vi "PDF Protokoll EPA1065_307.vi"(8 "error in (no error)":errorcluster caption="Fehler (Eingang, kein Fehler)") -> (0 "error out":errorcluster caption="Fehler (Ausgang)")   [LabVIEW 2020, in "Linearisierung v2.lvlib" / "Protokoll.lvlib"]
uses:
  Protokoll.lvlib
  EPA Ausgabetabelle.ctl
  AktivArray.ctl
  AktivButton.ctl
  Aktion Lin Daten aufarbeiten.ctl
  EPA1065-307/Aktion FGV Auswertung sammeln.ctl
  Seiten/FT-IR/FGV FT-IR Aktionen.ctl
  Seiten/System Einstellungen V2/Aktioen FGV System Konstanten.ctl
  Seiten/FT-IR/FGV FT-IR Gasliste Aktionen.ctl
  Seiten/System Einstellungen V2/Aktion FGV SystemEinstellungenV2.ctl
  Gasteiler/Aktionen FGV Gasteiler Daten.ctl
  <vilib>/Utility/miscctls.llb/LVPrintingMarginsTypeDef.ctl
  Linearisierung v2.lvlib
  EPA1065-307/Linearity verification 1065-307.lvlib
  Allgemein/allgemeine Sub-VIs.lvlib
  Seiten/FT-IR/FT-IR.lvlib
  Seiten/System Einstellungen V2/System Einstellungen V2.lvlib
  Gasteiler/Gasteiler.lvlib
panel:
  out "Serial number GT":string caption="Seriennummer:"
  out "Accuracy:":string caption="Genauigkeit:"
  out "Gas Bottle Nr.:":string caption="Gasflaschen Nr.:"
  out "Methode (Recipe):":string caption="Methode (Rezept):"
  out "Date & Time:":string caption="Datum & Zeit:"
  out "Versa Serial number:":string caption="Seriennummer:"
  out "Anlage:":string
  out "Serial number:":string caption="Seriennummer:"
  out "Messgerät:":string
  out "XY-Graph EPA":cluster{dbl[], dbl[]}[](graph) caption="XY-Graph"
  out "Aktiv":T1
  out "EPA Ausgabetabelle":T3
  out "Ergebnis:":string
  out "Konzentration:":string
  out "Komponente:":string
  out "Bearbeiter:":string
  out "Gasteiler:":string
  out "EPA Auswertung":string[][](table) caption="Evaluation"
  # "Linearity Check EPA § 1065.307"
  # "Linearity detection §1065.307"
  # "Description of the limits"
  # "Slope (a1) value between 0,99-1,01"
  # "Intercept (a0)"
  # "laboratory: Value <= 0,5% of the gas concentration"
  # "field: Value <= 1% of the gas concentration"
  # "Coefficient of determination (R²) Value >= 0,998"
  # "standard error of estimate (SEE) Value <= 1% of the gas concentration"
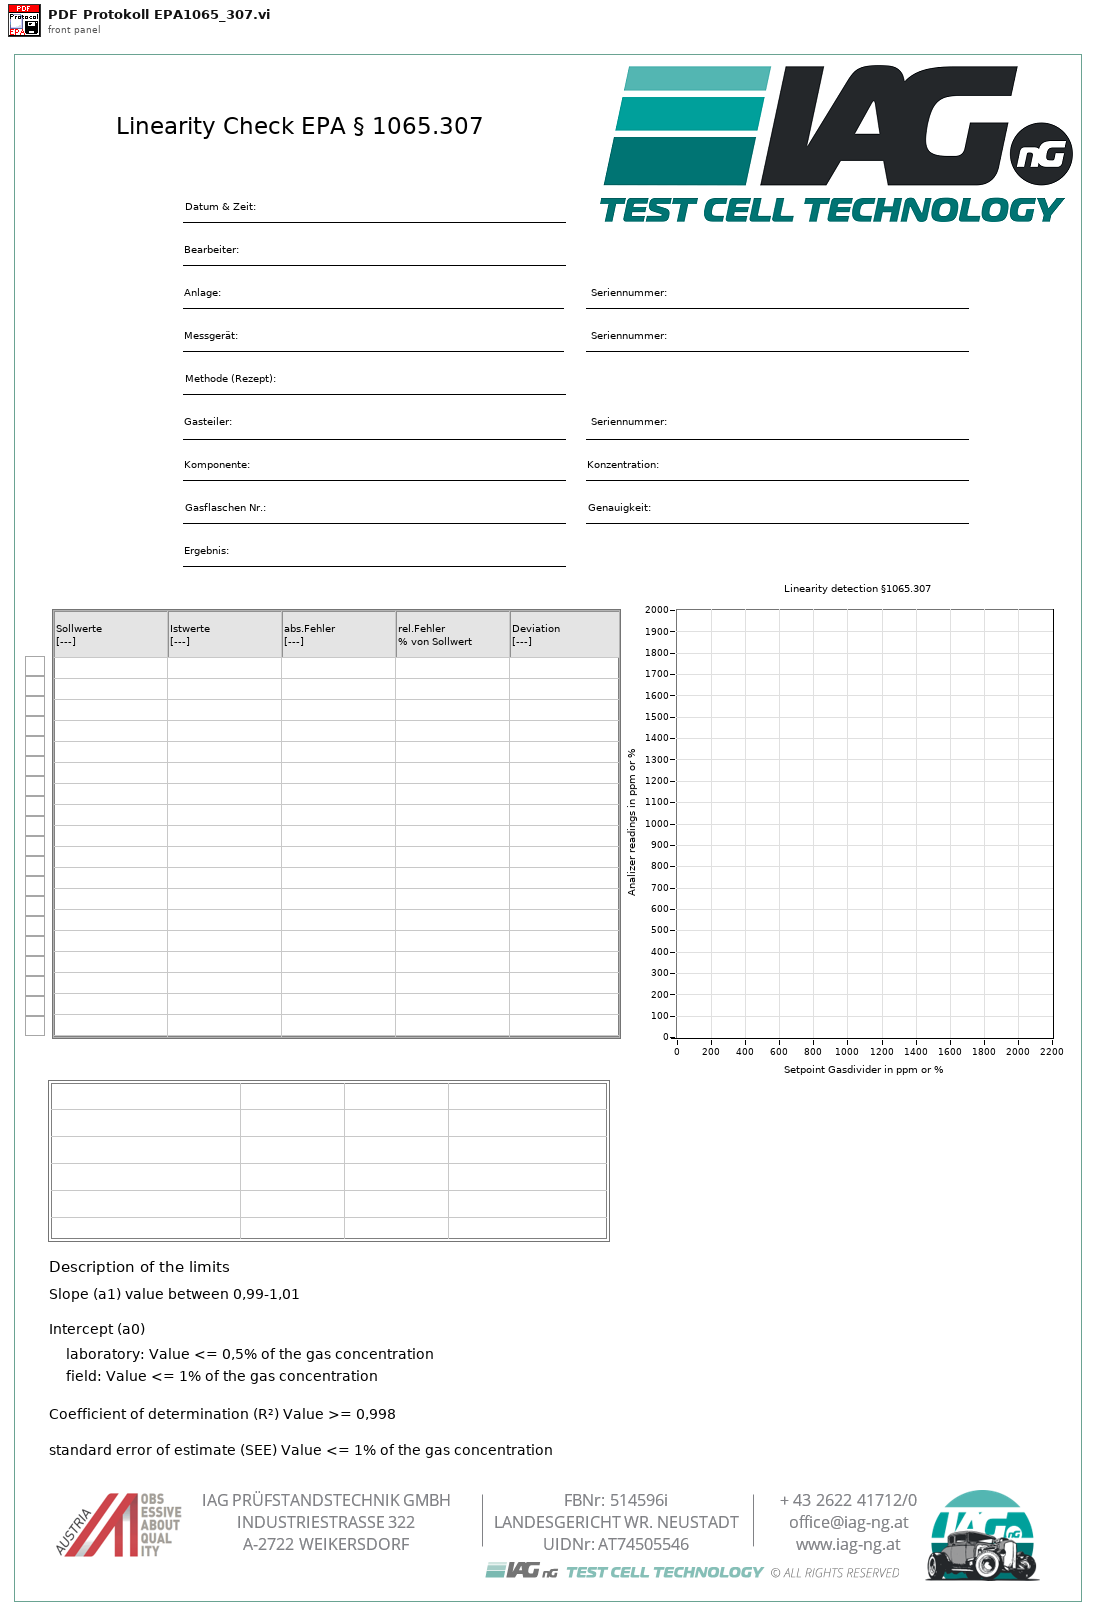
[diagram p1: front panel]
types:
  T1 = typedef "Linearisierung v2.lvlib/AktivArray.ctl" = T2[]
  T2 = typedef "Linearisierung v2.lvlib/AktivButton.ctl" = bool
  T3 = typedef "Linearisierung v2.lvlib/EPA Ausgabetabelle.ctl" = string[][]
  T4 = typedef "Linearisierung v2.lvlib/Gasteiler.lvlib/Aktionen FGV Gasteiler Daten.ctl" = enum16{"lesen", "Gasteiler Daten", "Seriellen Param.", "MB-Endwert", "laden", "speichern", "Anforderung", "TCP", "Aufzeichnung Start"}
  T5 = typedef "System Einstellungen V2.lvlib/Aktion FGV SystemEinstellungenV2.ctl" = enum16{"lesen", "Analysatoren schreiben", "Analysator ändern", "Analysatoren löschen", "laden", "speichern", "Untertitel", "Analysatoren", "Neue Analysatoren", "Gasteiler schreiben", "Gasteiler ändern", "Gasteiler löschen", "Gasteiler", "Gasteiler exportieren", "Gasteiler importieren"}
  T6 = typedef "FT-IR.lvlib/FGV FT-IR Gasliste Aktionen.ctl" = enum16{"lesen", "Gasliste FT-IR", "Gasliste ausgelesen", "laden", "speichern", "löschen"}
  T7 = typedef "System Einstellungen V2.lvlib/Aktioen FGV System Konstanten.ctl" = enum16{"lesen", "laden", "speichern", "Sprache"}
  T8 = typedef "FT-IR.lvlib/FGV FT-IR Aktionen.ctl" = enum16{"lesen", "NOG setzen", "NOS setzen", "Initialisieren", "speichern", "ALLES setzen", "FT-IR Spektrum loggen", "Komm Stoppen", "Spektrum LogKonfig"}
  T9 = typedef "Linearisierung v2.lvlib/Aktion Lin Daten aufarbeiten.ctl" = enum16{"lesen", "Protkolldaten", "speichern", "laden", "EPA auswerten", "Tabelle schreiben", "Lin auswerten", "Tab init", "Stufentabelle", "EPA aktiviert", "Nachbehandlung laden", "Tabelle löschen", "Istwerte löschen", "Zeile löschen", "Zeile einfügen", "LIN aktiviert", "LIN/EPA aktiv laden", "EGAK Tab", "LIN übernehmen", "Tab init ohne Stufen"}
  T10 = typedef "Linearisierung v2.lvlib/Linearity verification 1065-307.lvlib/Aktion FGV Auswertung sammeln.ctl" = enum16{"lesen", "Auswertung", "löschen"}
  T11 = enum32{"Portrait", "Landscape", "Rotated Portrait", "Rotated Landscape"}
  T12 = typedef "LVPrintingMarginsTypeDef.ctl" = cluster{"Top":sgl, "Left":sgl, "Bottom":sgl, "Right":sgl, "Measurement System":enum8{"Inches", "cm"}}
  T13 = cluster{"Modell":string, "ProjektNummer":string, "Software Version":string, "Seriennummer":string}
  T14 = typedef "Auswahlfeld.ctl" = u16
  T15 = typedef "Linearisierung v2.lvlib/Gasteiler.lvlib/Gasteiler Daten.ctl" = cluster{"Gasteiler":T16, "Gasteiler Stufen":T17, "Gasteiler Type":T18, "Konfig Gasteiler":T19, "Gasteiler Span Eingänge":u16}
  T16 = typedef "String - Eingabefeld.ctl" = string
  T17 = typedef "Linearisierung v2.lvlib/Gasteiler.lvlib/Gasteiler Stufen.ctl" = u16
  T18 = typedef "Linearisierung v2.lvlib/GasteilerType.ctl" = u16
  T19 = typedef "System Einstellungen V2.lvlib/Gasteiler Auswahl.ctl" = u16
  T20 = typedef "System Einstellungen V2.lvlib/Gasteiler.ctl" = cluster{"Gasteiler Name":string, "Gasteiler Type":string, "Gasteiler Seriennummer":string, "Gasteiler Letzte Wartung":timestamp}
  T21 = cluster{"GasteilerDefinitionsListe":T20[], "GasteilerDefinitionTextliste":string[][], "Gasteiler Strings And Values":cluster{"String":string, "Wert":string}[]}
  T22 = typedef "Linearisierung v2.lvlib/Eingabetabelle.ctl" = string[][]
  T23 = typedef "Linearisierung v2.lvlib/Lin-Polynom Daten.ctl" = cluster{"Messgerät":string, "Kalibrator (Gasteiler)":string, "Bearbeiter/in":string, "Komponente":string, "Zeitstempel":timestamp, "F_max gefordert (%)":sgl, "F_max in %":sgl, "F_max in ppm":sgl, "Vorschlag Ordnung":i32, "Polynom OK":bool, "Polynomkoeff.":dbl[], "Prüfgas Konzentration":dbl, "Pfad EPA":string, "Pfad_LIN":string, "Gasnummer:":u8, "Komponentenauswahl":T24, "Verdünnungsgas":T25, "Zeitdauer Stufe":T26, "Anzahl Stufen":T26, "F_max in % EPA":sgl, "F_max in ppm EPA":sgl, "F_max in % LIN":sgl, "F_max in ppm LIN":sgl, "Punkte umkehren":bool, "EPA Optionsfeld":T27, "Autolin Hovacal":T28, "Spanfactors":sgl[], "Kalibrierauswahl":T29, "Conditions:":T30, "Gasflaschen Nr.:":string, "Bottle Accuracy":dbl, "Konfig Gasflasche":T31, "Gasflasche":T32, "HovaCAL Flow AutoLin":T33, "MFC Output":T34, "Gas Ablaufdatum":timestamp, "Lin Modus":T35, "zusätzliche Zeitdauer Erster Punkt":sgl, "Offsets":sgl[]}
  T24 = typedef "Linearisierung v2.lvlib/KomponentenArray.ctl" = cluster{"Komponente:":T14, "Konzentration":dbl}[]
  T25 = typedef "Linearisierung v2.lvlib/Gasteiler.lvlib/Prüfgas in.ctl" = u16
  T26 = typedef "Zahlen-Eingabefeld.ctl" = sgl
  T27 = typedef "Linearisierung v2.lvlib/EPA Optionsfeld.ctl" = enum32{"Istwert", "Rohwert", "Linearisierter Wert"}
  T28 = typedef "Linearisierung v2.lvlib/Gasteiler.lvlib/HovaCal.lvlib/AutoLin Hovacal.ctl" = enum32{"Keine Auswahl", "Optionsauswahl 1", "Optionsauswahl 2"}
  T29 = typedef "Linearisierung v2.lvlib/Kalibrieroption.ctl" = u16
  T30 = typedef "Linearisierung v2.lvlib/Linearity verification 1065-307.lvlib/Condition.ctl" = u16
  T31 = typedef "System Einstellungen V2.lvlib/Konfig Gasflasche.ctl" = bool
  T32 = typedef "System Einstellungen V2.lvlib/Gasflasche Auswahl.ctl" = u16
  T33 = typedef "Linearisierung v2.lvlib/Gasteiler.lvlib/HovaCAL_Interface.lvlib/Controls.lvlib/Flow Einstellung.ctl" = cluster{"HovaCAL Flow Input Cluster":dbl}
  T34 = typedef "Linearisierung v2.lvlib/Gasteiler.lvlib/HovaCAL_Interface.lvlib/Controls.lvlib/Pump state.ctl" = cluster{"Run":bool}
  T35 = typedef "CalGas Aufschaltung.lvlib/Lin Modus.ctl" = u16
  T36 = typedef "String - Ausgabefeld.ctl" = string
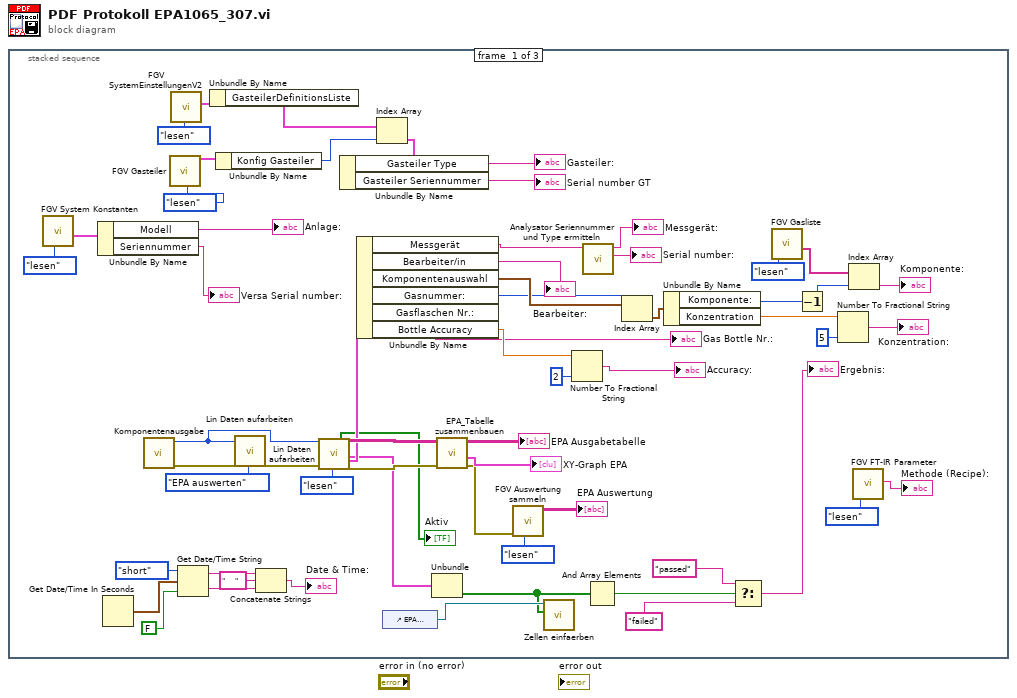
[diagram p0: block diagram]
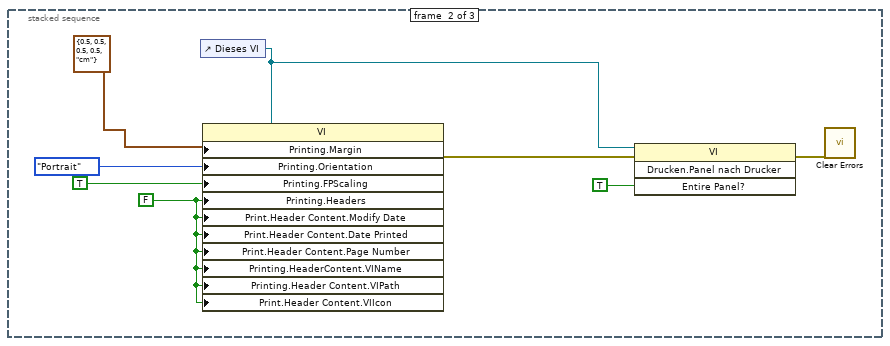
[diagram p2: hidden frame]
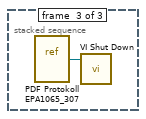
[diagram p3: hidden frame]
diagram:
  n1 = stacked-sequence {
    frame #0 {
      n2 = call "FGV System Konstanten.vi"("Aktionen"=Aktioen_FGV_System_Konstanten."lesen") -> ("Cluster out"=w21:T13)  [unwired: 6 in, 4 out]
      n3 = Unbundle By Name(w21) -> ("Modell"=→"Anlage:":string, "Seriennummer"=→"Versa Serial number:":string)
      n4 = Get Date/Time In Seconds() -> (seconds since 1Jan1904=w29:timestamp)
      n5 = call "Komponentenausgabe.vi"() -> ("error out"=w40:errorcluster, "Gaskomponente"=w39:T14)  [unwired: 8 in, 2 out]
      n6 = call "FGV Gasteiler.vi"("Aktionen"=Aktionen_FGV_Gasteiler_Daten."lesen") -> ("Gasteiler Daten"=w9:T15)  [unwired: 11 in, 7 out]
      n7 = call "FGV SystemEinstellungenV2.vi"("Aktion"=Aktion_FGV_SystemEinstellungenV2."lesen") -> ("Gasteiler"=w11:T21)  [unwired: 5 in, 5 out]
      n8 = Get Date/Time String(date format (0)=enum16{"short", "long", "abbreviated"}."short" ("Datumsformat (0)"), seconds (now)=w29, want seconds? (F)=FALSE ("Angabe von Sekunden? (F)")) -> (date string=w30:string, time string=w31:string)
      n9 = Unbundle By Name(w11) -> ("GasteilerDefinitionsListe"=w10:T20[])
      n10 = Unbundle By Name(w9) -> ("Konfig Gasteiler"=w7:T19)
      n11 = call "Lin Daten aufarbeiten.vi"("Index (Seite)"=w39, "error in (no error)"=w40, "Aktionen"=Aktion_Lin_Daten_aufarbeiten."EPA auswerten") -> ("error out"=w53:errorcluster)  [unwired: 14 in, 10 out]
      n12 = Concatenate Strings(w30, "     " ("String"), w31) -> (→"Date & Time:":string)
      n13 = call "Lin Daten aufarbeiten.vi"("Index (Seite)"=w39, "error in (no error)"=w53, "Aktionen"=Aktion_Lin_Daten_aufarbeiten."lesen") -> ("Aktiv EPA"=→"Aktiv":T1, "Eingabetabelle"=w61:T22, "EPA Auswertung"=w47:cluster{sgl[], sgl[], bool[]}, "Lin-Polynom"=w52:T23, "error out"=w60:errorcluster)  [unwired: 14 in, 6 out]
      n14 = Unbundle By Name(w52) -> ("Messgerät"=w13:string, "Bearbeiter/in"=→"Bearbeiter:":string, "Komponentenauswahl"=w50:T24, "Gasnummer:"=w49:u8, "Gasflaschen Nr.:"=→"Gas Bottle Nr.:":string, "Bottle Accuracy"=w24:dbl)
      n15 = Index Array(array=w10, index=w7) -> (element=w6:T20)
      n16 = Unbundle By Name(w6) -> ("Gasteiler Type"=→"Gasteiler:":string, "Gasteiler Seriennummer"=→"Serial number GT":string)
      n17 = control-ref of="EPA Auswertung"() -> (w37:refnum<vi>)
      n18 = Unbundle(w47) -> (w36:bool[])  [unwired: 2 out]
      n19 = call "EPA_Tabelle zusammenbauen.vi"("error in (no error)"=w60, "Eingabetabelle"=w61) -> ("error out"=w56:errorcluster, "XY-Graph"=→"XY-Graph EPA":cluster{dbl[], dbl[]}[], "EPA Ausgabetabelle"=→"EPA Ausgabetabelle":string[][])  [unwired: 7 in]
      n20 = call "FGV Auswertung sammeln.vi"("Aktion"=Aktion_FGV_Auswertung_sammeln."lesen", "error in (no error)"=w56) -> ("LINVer Auswertung"=→"EPA Auswertung":string[][])  [unwired: 7 in, 2 out]
      n21 = call "Zellen einfaerben.vi"("Färben"=w36, "Tabellenref."=w37) -> ()  [unwired: 10 in]
      n22 = Number To Fractional String(number=w24, precision (6)=i16 2 ("Genauigkeit (6)")) -> (F-format string=→"Accuracy:":string)  [unwired: 2 in]
      n23 = call "Analysator Seriennummer und Type ermitteln.vi"("Analysator"=w13) -> ("Type"=→"Serial number:":string, "Name für Protokoll"=→"Messgerät:":string)  [unwired: 8 in, 1 out]
      n24 = And Array Elements(Boolean array=w36) -> (logical AND=w35:bool)
      n25 = Index Array(array=w50, index=w49) -> (element=w48:cluster{"Komponente:":T14, "Konzentration":dbl})
      n26 = Unbundle By Name(w48) -> ("Komponente:"=w15:T14, "Konzentration"=w42:dbl)
      n27 = Select(t="passed", s=w35, f="failed") -> (s? t:f=→"Ergebnis:":string)
      n28 = call "FGV Gasliste.vi"("Aktionen"=FGV_FT-IR_Gasliste_Aktionen."lesen") -> ("Aktuelle Gasliste gesamt"=w3:T36[])  [unwired: 8 in, 2 out]
      n29 = Decrement(x=w15) -> (x-1=w14:T14)
      n30 = Number To Fractional String(number=w42, precision (6)=i16 5 ("Genauigkeit (6)")) -> (F-format string=→"Konzentration:":string)  [unwired: 2 in]
      n31 = Index Array(array=w3, index=w14) -> (element=→"Komponente:":T36)
      n32 = call "FGV FT-IR Parameter.vi"("Aktion"=FGV_FT-IR_Aktionen."lesen") -> ("Current Recipe"=→"Methode (Recipe):":string)  [unwired: 11 in, 7 out]
    }
    frame #1 {
      w66 = FALSE ("Drucken:Kopfzeilen?")
      n33 = control-ref of="Dieses VI"() -> (w63:refnum<vi>)
      n34 = property class="VI"(reference=w63, "Printing.Margin"=T12 {"Top"=0.5, "Left"=0.5, "Bottom"=0.5, "Right"=0.5, "Measurement System"=enum."cm"} ("Drucken:Ränder"), "Printing.Orientation"=T11."Portrait" ("Drucken:Seitenausrichtung"), "Printing.FPScaling"=TRUE ("Drucken:Frontpanel-Skalierung?"), "Printing.Headers"=w66, "Print.Header Content.Modify Date"=w66, "Print.Header Content.Date Printed"=w66, "Print.Header Content.Page Number"=w66, "Printing.HeaderContent.VIName"=w66, "Printing.Header Content.VIPath"=w66, "Print.Header Content.VIIcon"=w66) -> (error out=w70:errorcluster)  [unwired: 1 in, 1 out]
      n35 = invoke class="VI" method="Drucken.Panel nach Drucker"(reference=w63, error in=w70, "Entire Panel?"=TRUE ("Abschnittskopfzeilen?")) -> (error out=w64:errorcluster)  [unwired: 1 in, 3 out]
      n36 = call <vilib>:"Clear Errors.vi"("error in (no error)"=w64) -> ()  [unwired: 5 in, 2 out]
    }
    frame #2 {
      n37 = vi-ref "PDF Protokoll EPA1065_307.vi"() -> (w71:refnum<vi>)
      n38 = call "VI Shut Down.vi"("VI Referenz"=w71) -> ()  [unwired: 11 in]
    }
  }
